vi "Single Shot.vi"(8 "error in (no error)":errorcluster, 10 "mode (internal)":u16(ring) items=["internal", "external", "Q-switch"], 11 "Lotis in":refnum<class "PL Lotis TII LS.lvclass">) -> (0 "error out":errorcluster, 3 "Lotis out":refnum<class "PL Lotis TII LS.lvclass">)   [LabVIEW 2015, in "PL Lotis TII LS.lvclass"]
doc: "Single shot generation."
uses:
  PL Lotis TII LS.lvclass
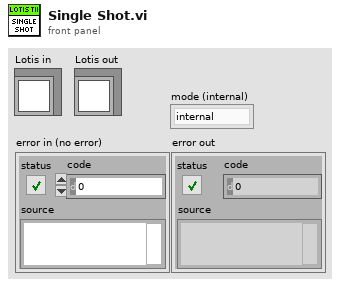
[diagram p1: front panel]
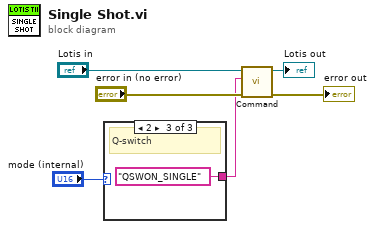
[diagram p0: block diagram]
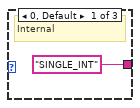
[diagram p2: hidden frame]
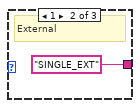
[diagram p3: hidden frame]
diagram:
  n1 = case shown="2" "mode (internal)" {
    tunnel: ["SINGLE_INT" ("command") "SINGLE_EXT" ("command") "QSWON_SINGLE" ("command")] -> w1
    frame 0, Default {
      # "Internal"
    }
    frame 1 {
      # "External"
    }
    frame 2 {
      # "Q-switch"
    }
  }
  n2 = call "Command.vi"("error in (no error)"="error in (no error)", "command"=w1, "Lotis in"="Lotis in") -> ("error out"=→"error out":errorcluster, "Lotis out"=→"Lotis out":refnum<class "PL Lotis TII LS.lvclass">)  [unwired: 6 in, 1 out]
